vi "U8 to U16.vi"(5 "次数":i32, 7 "data in":u8[](array[numeric])) -> (8 "data out":u16[](array[numeric]))   [LabVIEW 2016]
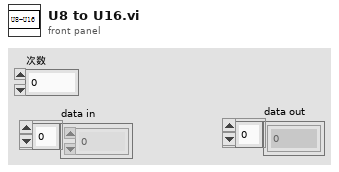
[diagram p1: front panel]
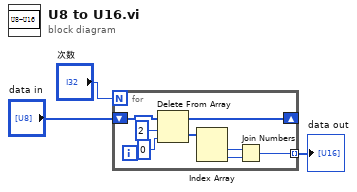
[diagram p0: block diagram]
diagram:
  n1 = for {
    N: "次数" -> [_]
    shift-right: [w11] -> _
    shift-left: "data in" -> [w5]
    tunnel: [w8] -> w2 mode=indexing
    n2 = Delete From Array(array=w5, length=2, index=0) -> (deleted portion=w4:u8[], array with subset deleted=w11:u8[])
    n3 = Index Array(array=w4) -> (element #1=w7:u8, element #2=w6:u8)  [unwired: 2 in]
    n4 = Join Numbers(hi=w7, lo=w6) -> ((hi.lo)=w8:u16)
  }
  "data out" <- w2
